vi "SetState.vi"(8 "Error In":errorcluster, 10 "State":bool, 11 "reference in":refnum<class "VdDigitalControl_AdvantechADAM.lvclass">) -> (0 "Error Out":errorcluster, 3 "reference out":refnum<class "VdDigitalControl_AdvantechADAM.lvclass">)   [LabVIEW 2020, in "VdDigitalControl_AdvantechADAM.lvclass"]
uses:
  VdDigitalControl_AdvantechADAM.lvclass
  VdDigitalControl_AdvantechADAM.lvclass/VdDigitalControl_AdvantechADAM.ctl
  VdDigitalControl_class/VdDigitalControl.lvclass
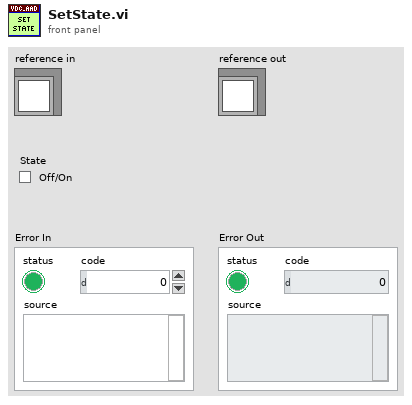
[diagram p1: front panel]
types:
  T1 = typedef "VdDigitalControl_AdvantechADAM.lvclass/ObjectAttributes.ctl" = cluster{"VISARef":refnum<visa-resource-name>}
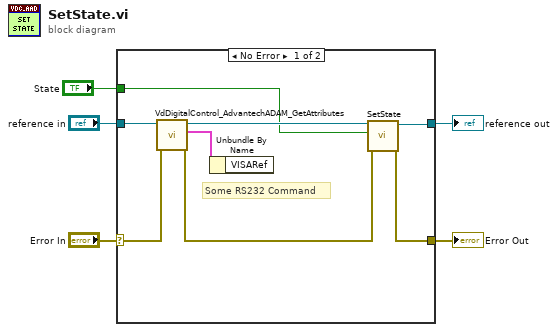
[diagram p0: block diagram]
diagram:
  n1 = case shown="No Error" "Error In" {
    selector: "Error In" -> [w7 w15]
    tunnel: [w9 w15] -> w4
    tunnel: [w10 w14] -> w2
    tunnel: "reference in" -> [w12 w14]
    tunnel: "State" -> [w8 _]
    frame No Error {
      # "Some RS232 Command"
      n2 = call "VdDigitalControl_AdvantechADAM_GetAttributes.vi"("error in"=w7, "reference in"=w12) -> ("error out"=w6:errorcluster, "Data"=w13:T1, "reference out"=w11:refnum<class "VdDigitalControl_AdvantechADAM.lvclass">)  [unwired: 6 in, 1 out]
      n3 = Unbundle By Name(w13) -> ()  [unwired: 1 out]
      n4 = call-parent "SetState.vi"("Error In"=w6, "State"=w8, "reference in"=w11) -> ("Error Out"=w9:errorcluster, "reference in"=w10:refnum<class "VdDigitalControl_AdvantechADAM.lvclass">)  [unwired: 7 in]
    }
    frame Error {
    }
  }
  "Error Out" <- w4
  "reference out" <- w2
